vi "GetRtd9219Properties.vi"(11 "Properties":T1[](array[typedef])) -> (0 "B":dbl, 1 "A":dbl, 2 "RTD type":u32, 3 "RTD ohm degree range":u32, 4 "C":dbl, 5 "Range/Mode":u32, 6 "r0":dbl)   [LabVIEW 2017, in "ScanEngine.lvlib"]
uses:
  <vilib>/addons/InsightCM/Devices/Shared/Common/ScanEngine/ScanEngine.lvlib
  <vilib>/addons/InsightCM/MessageBus/Base/controls/KeyValuePair.ctl
  <vilib>/addons/InsightCM/Utilities/PropertyHelpers/PropertyHelpers.lvlib
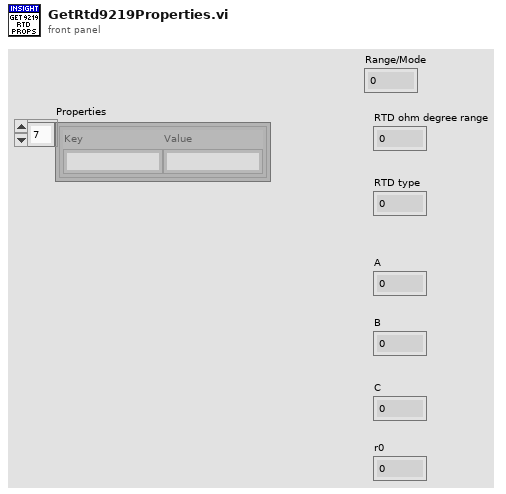
[diagram p1: front panel]
types:
  T1 = typedef "KeyValuePair.ctl" = cluster{"Key":string, "Value":string}
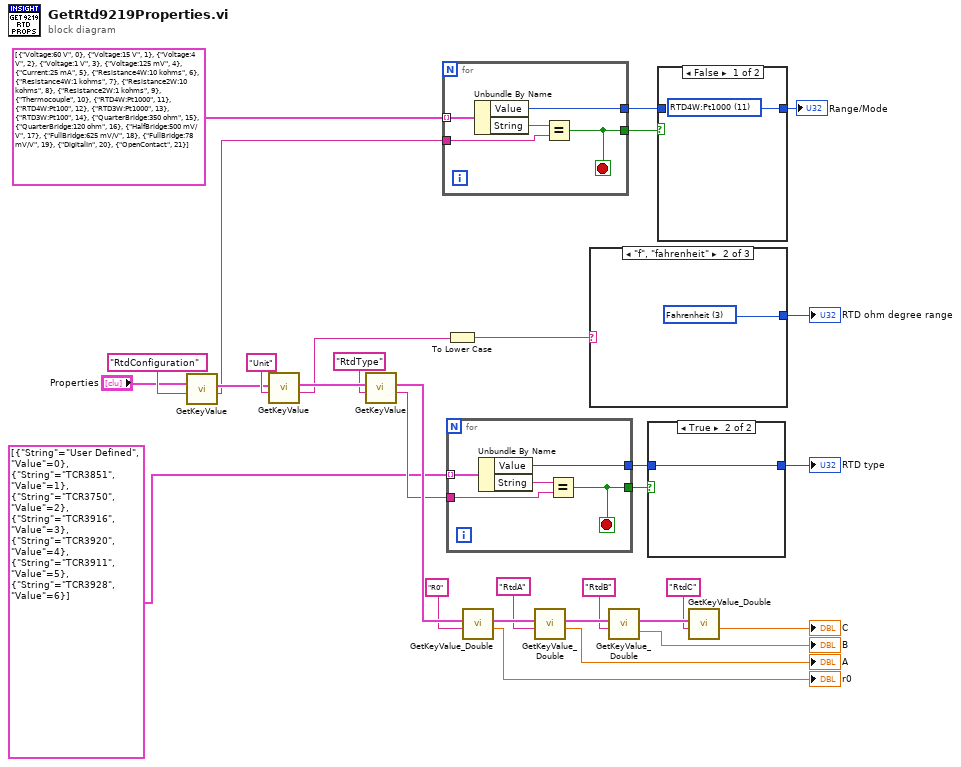
[diagram p0: block diagram]
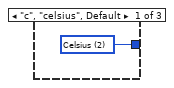
[diagram p2: hidden frame]
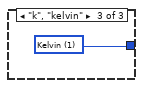
[diagram p3: hidden frame]
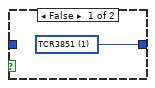
[diagram p5: hidden frame]
diagram:
  n1 = call <vilib>:"GetKeyValue.vi"("key"="RtdConfiguration" ("name"), "key value pairs"="Properties") -> ("value"=w9:string, "key value pairs out"=w10:T1[])  [unwired: 7 in, 1 out]
  n2 = call <vilib>:"GetKeyValue.vi"("key"="Unit" ("name"), "key value pairs"=w10) -> ("value"=w4:string, "key value pairs out"=w28:T1[])  [unwired: 7 in, 1 out]
  n3 = call <vilib>:"GetKeyValue.vi"("key"="RtdType" ("name"), "key value pairs"=w28) -> ("value"=w17:string, "key value pairs out"=w27:T1[])  [unwired: 7 in, 1 out]
  n4 = for {
    tunnel: cluster{"String":string, "Value":u32}[] [{"String"="Voltage:60 V", "Value"=0}, {"String"="Voltage:15 V", "Value"=1}, {"String"="Voltage:4 V", "Value"=2}, {"String"="Voltage:1 V", "Value"=3}, {"String"="Voltage:125 mV", "Value"=4}, {"String"="Current:25 mA", "Value"=5}, {"String"="Resistance4W:10 kohms", "Value"=6}, {"String"="Resistance4W:1 kohms", "Value"=7}, {"String"="Resistance2W:10 kohms", "Value"=8}, {"String"="Resistance2W:1 kohms", "Value"=9}, {"String"="Thermocouple", "Value"=10}, {"String"="RTD4W:Pt1000", "Value"=11}, {"String"="RTD4W:Pt100", "Value"=12}, {"String"="RTD3W:Pt1000", "Value"=13}, {"String"="RTD3W:Pt100", "Value"=14}, {"String"="QuarterBridge:350 ohm", "Value"=15}, {"String"="QuarterBridge:120 ohm", "Value"=16}, {"String"="HalfBridge:500 mV/V", "Value"=17}, {"String"="FullBridge:625 mV/V", "Value"=18}, {"String"="FullBridge:78 mV/V", "Value"=19}, {"String"="DigitalIn", "Value"=20}, {"String"="OpenContact", "Value"=21}] ("Strings And Values []") -> [w36] mode=indexing
    tunnel: [w34] -> w7
    tunnel: w9 -> [w33]
    tunnel: [w32] -> w8
    stop <- w32 stop-if-true
    n5 = Unbundle By Name(w36) -> ("Value"=w34:u32, "String"=w35:string)
    n6 = Equal?(x=w35, y=w33) -> (x = y?=w32:bool)
  }
  n7 = To Lower Case(string=w4) -> (all lower case string=w3:string)
  n8 = for {
    tunnel: cluster{"String":string, "Value":u32}[] [{"String"="User Defined", "Value"=0}, {"String"="TCR3851", "Value"=1}, {"String"="TCR3750", "Value"=2}, {"String"="TCR3916", "Value"=3}, {"String"="TCR3920", "Value"=4}, {"String"="TCR3911", "Value"=5}, {"String"="TCR3928", "Value"=6}] ("Strings And Values []") -> [w41] mode=indexing
    tunnel: [w39] -> w31
    tunnel: w17 -> [w38]
    tunnel: [w37] -> w30
    stop <- w37 stop-if-true
    n9 = Unbundle By Name(w41) -> ("Value"=w39:u32, "String"=w40:string)
    n10 = Equal?(x=w40, y=w38) -> (x = y?=w37:bool)
  }
  n11 = call <vilib>:"GetKeyValue_Double.vi"("key"="R0" ("name"), "key value pairs"=w27) -> ("value"=→"r0":dbl, "key value pairs out"=w26:T1[])  [unwired: 7 in, 1 out]
  n12 = call <vilib>:"GetKeyValue_Double.vi"("key"="RtdA" ("name"), "key value pairs"=w26) -> ("value"=→"A":dbl, "key value pairs out"=w25:T1[])  [unwired: 7 in, 1 out]
  n13 = case shown="\"f\", \"fahrenheit\"" w3 {
    tunnel: [w42 w43 w44] -> w5
    frame "c", "celsius", Default {
      w42 = u32 2 items=["Ohms", "Kelvin", "Celsius", "Fahrenheit", "Rankine"] ("RTD0:Ohm degree range")
    }
    frame "f", "fahrenheit" {
      w43 = u32 3 items=["Volts", "Kelvin", "Celsius", "Fahrenheit", "Rankine"] ("CH3:Degree range")
    }
    frame "k", "kelvin" {
      w44 = u32 1 items=["Volts", "Kelvin", "Celsius", "Fahrenheit", "Rankine"] ("CH3:Degree range")
    }
  }
  "RTD ohm degree range" <- w5
  n14 = call <vilib>:"GetKeyValue_Double.vi"("key"="RtdB" ("name"), "key value pairs"=w25) -> ("value"=→"B":dbl, "key value pairs out"=w24:T1[])  [unwired: 7 in, 1 out]
  n15 = case shown="True" w30 {
    tunnel: [w45 w46] -> w29
    tunnel: w31 -> [_ w46]
    frame False {
      w45 = u32 1 items=["User Defined", "TCR3851", "TCR3750", "TCR3916", "TCR3920", "TCR3911", "TCR3928"] ("RTD0:RTD type")
    }
    frame True {
    }
  }
  "RTD type" <- w29
  n16 = case shown="False" w8 {
    tunnel: [w47 w48] -> w6
    tunnel: w7 -> [_ w48]
    frame False {
      w47 = u32 11 items=["Voltage:60 V", "Voltage:15 V", "Voltage:4 V", "Voltage:1 V", "Voltage:125 mV", "Current:25 mA", "Resistance4W:10 kohms", "Resistance4W:1 kohms", "Resistance2W:10 kohms", "Resistance2W:1 kohms", "Thermocouple", "RTD4W:Pt1000", "RTD4W:Pt100", "RTD3W:Pt1000", "RTD3W:Pt100", "QuarterBridge:350 ohm", "QuarterBridge:120 ohm", "HalfBridge:500 mV/V", "FullBridge:625 mV/V", "FullBridge:78 mV/V", "DigitalIn", "OpenContact"] ("CH3:Range / Mode")
    }
    frame True {
    }
  }
  "Range/Mode" <- w6
  n17 = call <vilib>:"GetKeyValue_Double.vi"("key"="RtdC" ("name"), "key value pairs"=w24) -> ("value"=→"C":dbl)  [unwired: 7 in, 2 out]
